vi "Configure DC Volts.vi"(5 "AutoZero":u16(ring)=1 items=["OFF", "ON", "ONCE"], 6 "AutoDelay":u16(ring) items=["OFF", "ON", "ONCE"], 7 "NPLC":dbl=1.0 min=0.001 max=10.0, 8 "error in":errorcluster, 9 "Range (1.000)":dbl=1.0, 10 "AutoRange  On":bool, 11 "VISA resource name":refnum<visa-resource-name>) -> (0 "error out":errorcluster, 3 "VISA resource name out":refnum<visa-resource-name>, 4 "Command String":string)   [LabVIEW 2018, in "Keithley 3706.lvlib"]
uses:
  <instrlib>/Keithley 3706/Keithley 3706.lvlib
panel:
  # "V"
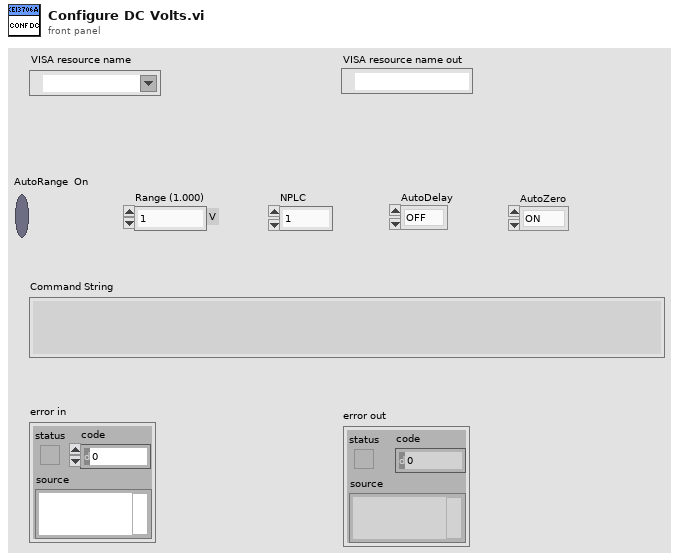
[diagram p1: front panel]
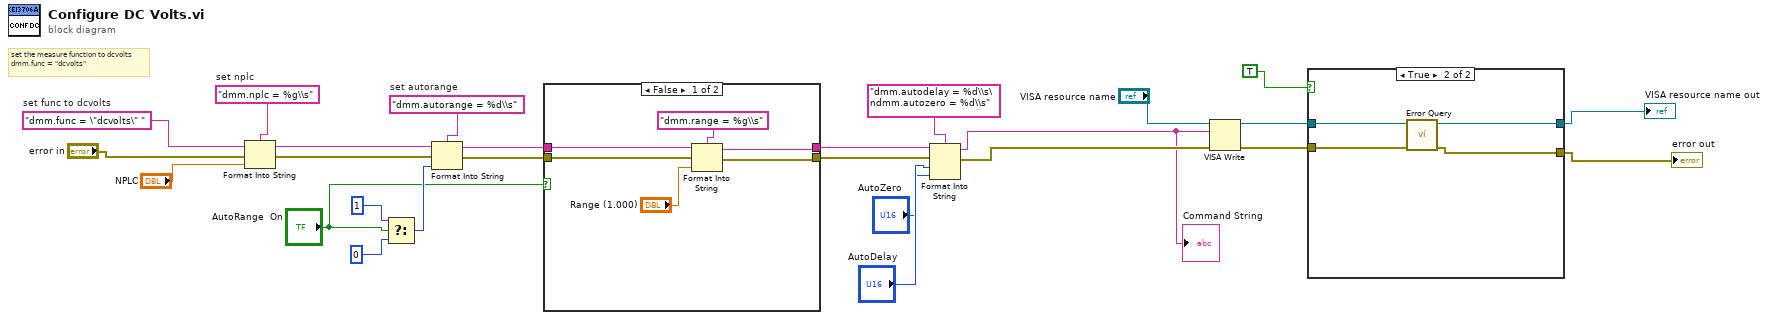
[diagram p0: block diagram]
diagram:
  w20 = "dmm.autorange = %d\\s"  # set autorange
  w23 = "dmm.nplc = %g\\s"  # set nplc
  w26 = "dmm.func = \"dcvolts\" "  # set func to dcvolts
  # "set the measure function to dcvolts\ndmm.func = \"dcvolts\""
  n1 = Format Into String(format string=w23, initial string=w26, error in="error in", "NPLC") -> (resulting string=w22:string, error out=w21:errorcluster)
  n2 = Select(t=1, s="AutoRange  On", f=0) -> (s? t:f=w17:i32)
  n3 = Format Into String(format string=w20, initial string=w22, error in=w21, w17) -> (resulting string=w15:string, error out=w14:errorcluster)
  n4 = case shown="False" "AutoRange  On" {
    tunnel: w15 -> [w32 w34]
    tunnel: w14 -> [w31 w33]
    tunnel: [w28 w34] -> w13
    tunnel: [w27 w33] -> w12
    frame False {
      n5 = Format Into String(format string="dmm.range = %g\\s", initial string=w32, error in=w31, "Range (1.000)") -> (resulting string=w28:string, error out=w27:errorcluster)
    }
    frame True {
    }
  }
  n6 = Format Into String(format string="dmm.autodelay = %d\\s\ndmm.autozero = %d\\s", initial string=w13, error in=w12, "AutoDelay", "AutoZero") -> (resulting string=w3:string, error out=w10:errorcluster)
  "Command String" <- w3
  n7 = VISA Write(VISA resource name="VISA resource name", write buffer=w3, error in (no error)=w10) -> (VISA resource name out=w7:refnum<visa-resource-name>, error out=w6:errorcluster)  [unwired: 1 out]
  n8 = case shown="True" TRUE {
    tunnel: w7 -> [w36 w40]
    tunnel: w6 -> [w35 w39]
    tunnel: [w36 w38] -> w5
    tunnel: [w35 w37] -> w4
    frame False {
    }
    frame True {
      n9 = call <instrlib>:"Error Query.vi"("error in (no error)"=w39, "VISA resource name"=w40) -> ("error out"=w37:errorcluster, "VISA resource name output"=w38:refnum<visa-resource-name>)  [unwired: 6 in, 2 out]
    }
  }
  "VISA resource name out" <- w5
  "error out" <- w4
